vi "AssignColors.vi"(6 "Add Spaces?":bool, 11 "Code":refnum<vi>) -> (2 "Value":string)   [LabVIEW 2020]
uses:
  <vilib>/Utility/miscctls.llb/LVSelectionTypeDef.ctl
  ColorGlobals.vi
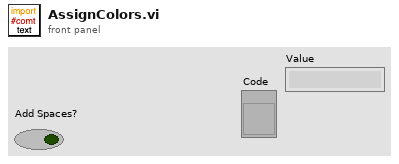
[diagram p1: front panel]
types:
  T1 = typedef "LVSelectionTypeDef.ctl" = cluster{"Selection Start":u32, "Selection End":u32}
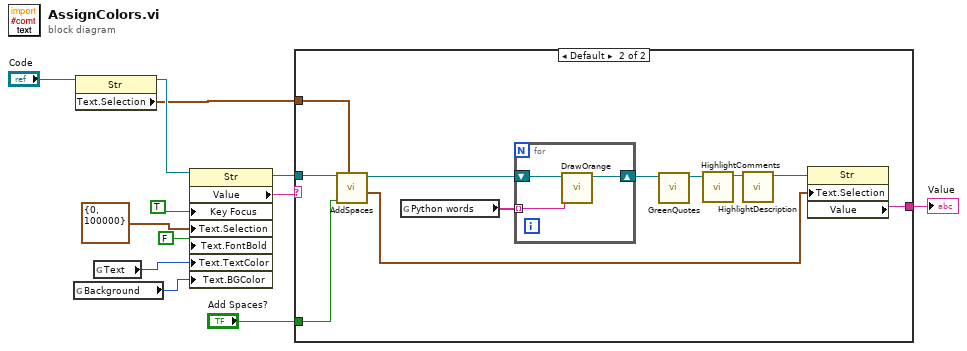
[diagram p0: block diagram]
diagram:
  n1 = global read "ColorGlobals.vi" "Background"() -> (w1:u32)
  n2 = property on="Property Node" class="Str"(reference="Code") -> (reference out=w9:refnum<vi>, "Text.Selection"=w8:T1)  [unwired: 1 in, 1 out]
  n3 = global read "ColorGlobals.vi" "Text"() -> (w2:u32)
  n4 = property on="Property Node" class="Str"(reference=w9, "Key Focus"=TRUE, "Text.Selection"=T1 {"Selection Start"=0, "Selection End"=100000}, "Text.FontBold"=FALSE ("Text.Font:Bold"), "Text.TextColor"=w2, "Text.BGColor"=w1) -> (reference out=w4:refnum<vi>, "Value"=w3:string)  [unwired: 1 in, 1 out]
  n5 = case shown="Default" w3 {
    selector: w3 -> [w13 _]
    tunnel: w4 -> [_ w20]
    tunnel: w8 -> [_ w24]
    tunnel: [w13 w23] -> w6
    tunnel: "Add Spaces?" -> [_ w21]
    frame "" {
    }
    frame Default {
      n6 = call "AddSpaces.vi"("Text.Selection"=w24, "Add Spaces?"=w21, "String in"=w20) -> ("Cursor"=w22:cluster{u32, u32}, "String out"=w19:refnum<vi>)  [unwired: 7 in]
      n7 = global read "ColorGlobals.vi" "Python words"() -> (w14:string[])
      n8 = for {
        shift-right: [w26] -> w15
        shift-left: w19 -> [w27]
        tunnel: w14 -> [w25] mode=indexing
        n9 = call "DrawOrange.vi"("Expression"=w25, "String in"=w27) -> ("String out"=w26:refnum<vi>)  [unwired: 9 in]
      }
      n10 = call "GreenQuotes.vi"("String in"=w15) -> ("String out"=w16:refnum<vi>)  [unwired: 10 in]
      n11 = call "HighlightComments.vi"("String in"=w16) -> ("String out"=w17:refnum<vi>)  [unwired: 10 in]
      n12 = call "HighlightDescription.vi"("String in"=w17) -> ("String out"=w18:refnum<vi>)  [unwired: 10 in]
      n13 = property on="Property Node" class="Str"(reference=w18, "Text.Selection"=w22) -> ("Value"=w23:string)  [unwired: 1 in, 2 out]
    }
  }
  "Value" <- w6
